vi "TagDB-TestMain(inside).vi"() -> ()   [LabVIEW 2017, in "tagdb-tester.lvlib"]
uses:
  tagdb-tester.lvlib
  7a71b126-9f55-4317-a22e-de5e26c405bb.vi
  0b4a98d8-f064-4be9-924c-5f06de3aa089.vi
  src/TagDB/_Support/DataAccess/_NameCacher.vi
  src/TagDB/_Support/Error/_[error50002]Invalid DataType.vi
  src/TagDB/_Support/Error/_[error50000]Invalid DB REF.vi
  src/TagDB/_Support/DataAccess/TagDB Ref to DVR.vi
  src/TagDB/_Support/URL/TRIM-BOTH-SPACE.vi
  src/TagDB/_Support/DataAccess/data-Write.vi
  src/TagDB/_Support/DataAccess/_datatypeChecker.vi
  <vilib>/Utility/Data Type/Get Type Information.vi
  src/TagDB/_Support/Error/_Build Error Cluster.vi
  src/TagDB/TagDB.lvlib
panel:
  in  "stop":bool
  out "Value":variant
  in  "read tag":string="abc"
  in  "Numeric":i32=123124312
  in  "write tag":string="abc"
  in  "name (unnamed)":string="db"
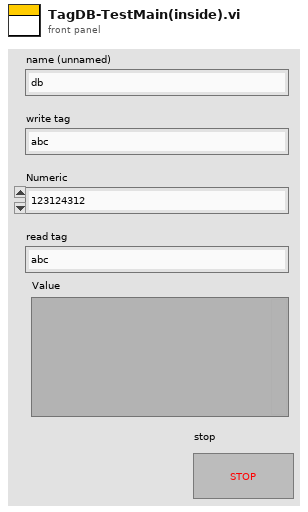
[diagram p1: front panel]
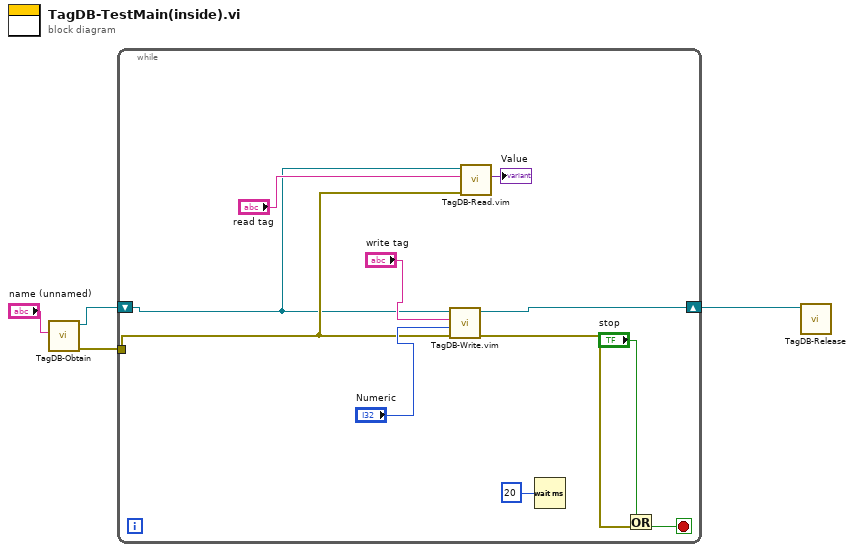
[diagram p0: block diagram]
diagram:
  n1 = call "TagDB-Obtain.vi"("name (unnamed)"="name (unnamed)") -> ("error out"=w4:errorcluster, "TagDB"=w3:refnum<k1>)  [unwired: 4 in, 1 out]
  n2 = while {
    tunnel: w4 -> [w10]
    shift-right: [w13] -> w1
    shift-left: w3 -> [w9]
    stop <- w6 stop-if-true
    n3 = call "TagDB-Write.vim"("error in (no error)"=w10, "Value"="Numeric", "tag"="write tag", "TagDB"=w9) -> ("error out"=w12:errorcluster, "TagDB(dup)"=w13:refnum<k1>)  [unwired: 5 in, 1 out]
    n4 = call "TagDB-Read.vim"("error in (no error)"=w10, "name"="read tag", "TagDB"=w9) -> ("Value"=→"Value":variant)  [unwired: 3 in, 5 out]
    n5 = Wait (ms)(milliseconds to wait=u32 20 ("millisecond timer value")) -> ()  [unwired: 1 out]
    n6 = Or(x="stop", y=w12) -> (x .or. y?=w6:bool)
  }
  n7 = call "TagDB-Release.vi"("TagDB"=w1) -> ()  [unwired: 10 in, 1 out]
